vi "Play.vi"(8 "error in (no error)":errorcluster, 10 "Sound":refnum<class "Sound.lvclass">=refnum, 11 "Sound Card":refnum<class "Sound Card.lvclass">) -> (0 "error out":errorcluster, 3 "Sound Player out":refnum<class "Sound Card.lvclass">)   [LabVIEW 2010, in "Sound Card.lvclass"]
doc: "Play a sound on the Sound Card."
uses:
  Sound Card.lvclass
  Sound/Sound.lvclass
  Sound Card.lvclass/Sound Card.ctl
  <vilib>/sound2/lvsound2.llb/Sound Output Write (DBL).vi
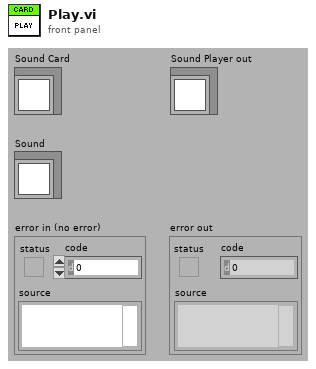
[diagram p1: front panel]
types:
  T1 = typedef "Sound Output Task ID.ctl" = u32
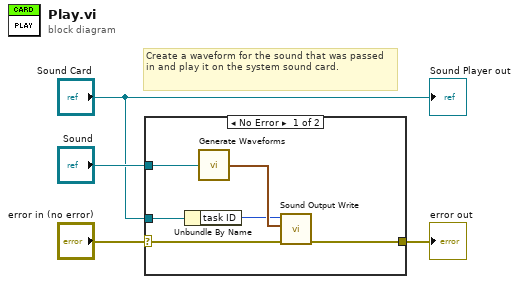
[diagram p0: block diagram]
diagram:
  # "Create a waveform for the sound that was passed in and play it on the system sound card."
  n1 = case shown="No Error" "error in (no error)" {
    selector: "error in (no error)" -> [w6 w11]
    tunnel: [w5 w11] -> w3
    tunnel: "Sound" -> [w10 _]
    tunnel: "Sound Card" -> [w8 _]
    frame No Error {
      n2 = Unbundle By Name(w8) -> ("task ID"=w7:T1)
      n3 = call-dynamic "Generate Waveforms.vi"("Sound.lvclass"=w10) -> ("Waveforms"=w9:waveform(dbl)[])
      n4 = call-poly <vilib>:"Sound Output Write.vi"("error in (no error)"=w6, "data"=w9, "task ID"=w7) -> ("error out"=w5:errorcluster)  [unwired: 7 in, 1 out]
    }
    frame Error {
    }
  }
  "error out" <- w3
  "Sound Player out" <- "Sound Card"
